vi "search_cv.vi"(10 "data":map{i32, T1}(c390)) -> ()   [LabVIEW 2024, in "CLZ_to_ComicVine.lvlib"]
uses:
  comic_manager/manager_daemon/type_defs/VolumeData--cluster.ctl
  CV_Shared_Library/volume.type--enum.ctl
  CLZ_to_ComicVine.lvlib
  <userlib>/_OpenG.lib/string/string.llb/openg_string.lvlib
  CV_Shared_Library/CV_Shared_Library.lvlib
  comic_manager/manager_daemon/manager_daemon.lvclass
panel:
  out "search results":string[](array[string])
  in  "trim string":string=", vol"
  in  "search value":string
  in  "Array in":string[](array[string])
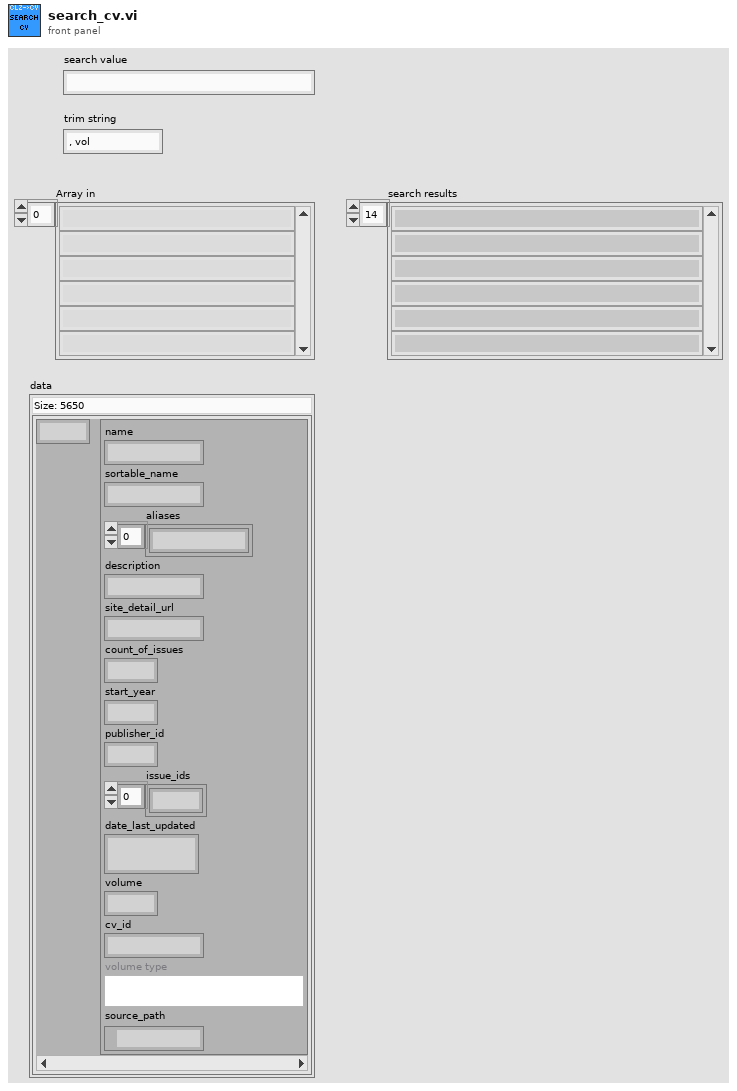
[diagram p1: front panel]
types:
  T1 = typedef "manager_daemon.lvclass/VolumeData--cluster.ctl" = cluster{"name":string, "sortable_name":string, "aliases":string[], "description":string, "site_detail_url":string, "count_of_issues":i32, "start_year":i32, "publisher_id":i32, "issue_ids":i32[], "date_last_updated":timestamp, "volume":i32, "cv_id":string, "volume type":T2, "source_path":path}
  T2 = typedef "CV_Shared_Library.lvlib/volume.type--enum.ctl" = enum16{"Ongoing", "Limited Series", "Annual", "One Shot", "Reprint/Document", "Star Comics", "Epic Comics"}
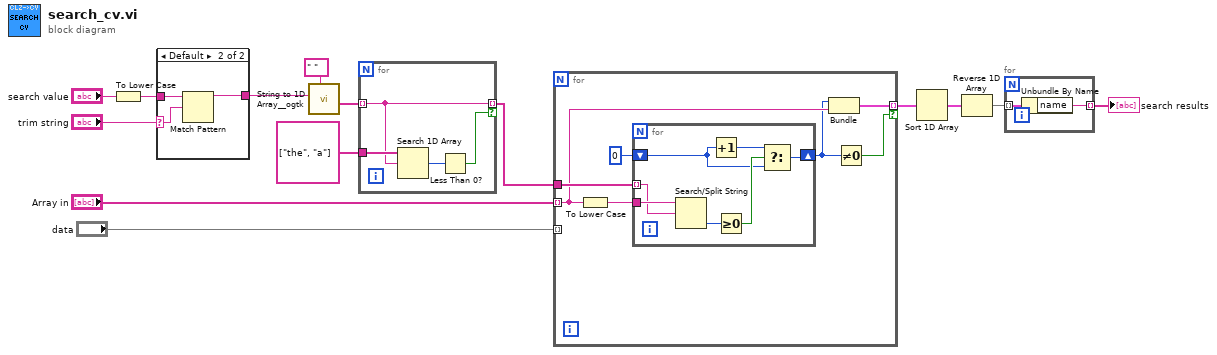
[diagram p0: block diagram]
diagram:
  n1 = To Lower Case(string="search value") -> (all lower case string=w11:string)
  n2 = case shown="Default" "trim string" {
    selector: "trim string" -> [_ w17]
    tunnel: w11 -> [w15 w18]
    tunnel: [w15 w16] -> w9
    frame "" {
    }
    frame Default {
      n3 = Match Pattern(string=w18, regular expression=w17) -> (before substring=w16:string)  [unwired: 1 in, 3 out]
    }
  }
  n4 = call <userlib>:"String to 1D Array__ogtk.vi"("delimiter (Tab)"=" ", "string"=w9) -> ("Array of Strings"=w12:string[])  [unwired: 9 in]
  n5 = for {
    tunnel: w12 -> [w21] mode=indexing
    tunnel: string[] ["the", "a"] -> [w22]
    tunnel: [w21] -> w6 mode=indexing if=w19
    n6 = Search 1D Array(1D array=w22, element=w21) -> (index of element=w20:i32)  [unwired: 1 in]
    n7 = Less Than 0?(x=w20) -> (x < 0?=w19:bool)
  }
  n8 = for {
    tunnel: "Array in" -> [w27] mode=indexing
    tunnel: w6 -> [w29]
    tunnel: [w26] -> w5 mode=indexing if=w24
    tunnel: "data" -> [_] mode=indexing
    n9 = To Lower Case(string=w27) -> (all lower case string=w23:string)
    n10 = for {
      tunnel: w29 -> [w35] mode=indexing
      tunnel: w23 -> [w36]
      shift-right: [w30] -> w25
      shift-left: 0 -> [w32]
      n11 = Search/Split String(string=w36, search string/char (-)=w35) -> (offset of match=w34:i32)  [unwired: 1 in, 2 out]
      n12 = Increment(x=w32) -> (x+1=w31:i32)
      n13 = Greater Or Equal To 0?(x=w34) -> (x >= 0?=w33:bool)
      n14 = Select(t=w31, s=w33, f=w32) -> (s? t:f=w30:i32)
    }
    n15 = Bundle(w25, "name"=w27) -> (w26:cluster{i32, "name":string})  [unwired: 1 in]
    n16 = Not Equal To 0?(x=w25) -> (x != 0?=w24:bool)
  }
  n17 = Sort 1D Array(array=w5) -> (sorted array=w4:cluster{i32, "name":string}[])
  n18 = Reverse 1D Array(array=w4) -> (reversed array=w3:cluster{i32, "name":string}[])
  n19 = for {
    tunnel: w3 -> [w38] mode=indexing
    tunnel: [w37] -> w2 mode=indexing
    n20 = Unbundle By Name(w38) -> ("name"=w37:string)
  }
  "search results" <- w2
